vi "Simu_Temp.vi"(1 "Lmax":dbl, 2 "Lmin":dbl) -> (0 "Numeric":dbl)   [LabVIEW 2020]
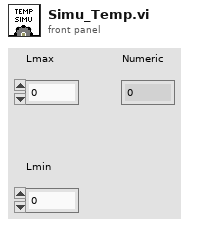
[diagram p1: front panel]
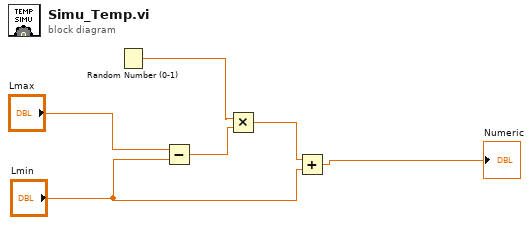
[diagram p0: block diagram]
diagram:
  n1 = Random Number (0-1)() -> (number: 0 to 1=w2:dbl)
  n2 = Subtract(x="Lmax", y="Lmin") -> (x-y=w3:dbl)
  n3 = Multiply(x=w2, y=w3) -> (x*y=w4:dbl)
  n4 = Add(x=w4, y="Lmin") -> (x+y=→"Numeric":dbl)
